vi "IFC.vi"(0 "System no.":i32=1 min=1 step=1, 2 "Interface parameter":string[](array[string]), 3 "Parameter value":string[](array[string]), 5 "error in":errorcluster) -> (19 "error out":errorcluster)   [LabVIEW 2026]
doc: "Changes the current interface configuration. After IFC is sent, the new interface configuration of the controller becomes active and the host must change the interface configuration too. Settings made with IFC are valid until the controller is powered down. \nTo save them to EPROM and make them the default use IFS instead.\n\nC-884: MACADR cannot be changed with IFC. To change IPADR the use of IFS is recommended instead. \n\nC-885: MACADR cannot be changed with IFC. To change IPADR the use of IFS is recommended instead.\n\nE-517: The current active RS-232 baud rate and GPIB (IEEE 488) address can also be set on the E-517 front panel in the COMMUNICATION display screen. This screen can be accessed by the trackball. The front panel settings interdepend with the interface parameter settings set with IFC. See E-517 user manual for details.\n\nE-709: Use IFC to change baud rate settings only.\n\nE-712, E-725, E-727, E-753, E-754, E-871, E-872, E-873, E-874: Use IFC to change baud rate settings only, for all other settings use IFS instead."
panel:
  # "Changes the current InterFace Configuration. After IFC is sent, the new interface\nconfiguration of the controller becomes active and the host must change the interface\nconfiguration too. Settings made with IFC are valid until the controller is powered down. \nTo save them to EPROM and make them the default use IFS instead."
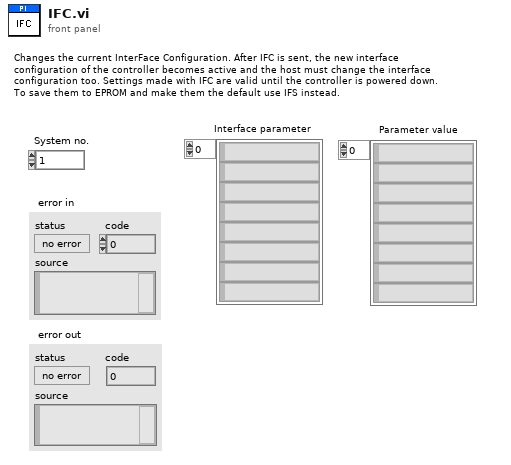
[diagram p1: front panel]
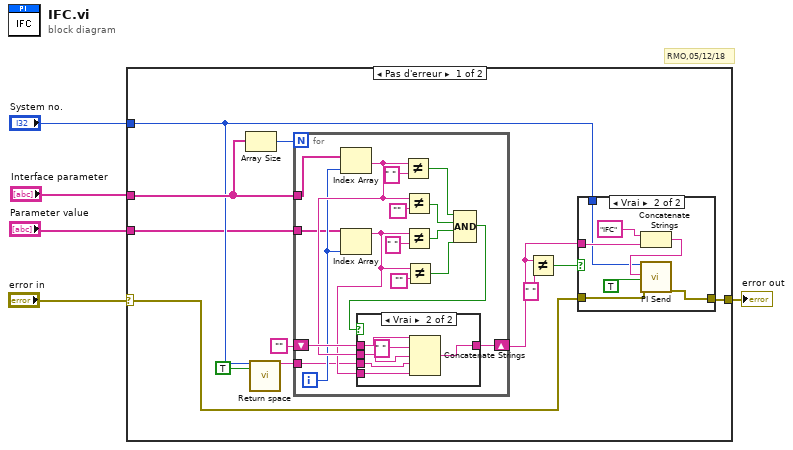
[diagram p0: block diagram]
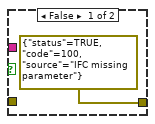
[diagram p2: hidden frame]
diagram:
  # "RMO,05/12/18"
  n1 = case shown="Pas d'erreur" "error in" {
    selector: "error in" -> [w6 w50]
    tunnel: "Interface parameter" -> [w17 _]
    tunnel: [w8 w50] -> w4
    tunnel: "Parameter value" -> [w15 _]
    tunnel: "System no." -> [w16 _]
    frame No Error {
      n2 = Array Size(array=w17) -> (size(s)=w10:i32)
      n3 = call "Return space.vi"("System no."=w16, "With space?"=TRUE) -> ("String out"=w9:string)  [unwired: 17 out]
      n4 = for {
        N: w10 -> [_]
        tunnel: w17 -> [w31]
        shift-right: [w40] -> w12
        shift-left: "" -> [w41]
        tunnel: w15 -> [w29]
        tunnel: w9 -> [w26]
        i -> [w30]
        n5 = Index Array(array=w31, index=w30) -> (element=w39:string)
        n6 = Index Array(array=w29, index=w30) -> (element=w28:string)
        n7 = Not Equal?(x=w39, y=" ") -> (x != y?=w35:bool)
        n8 = Not Equal?(x=w39, y="") -> (x != y?=w34:bool)
        n9 = Not Equal?(x=w28, y=" ") -> (x != y?=w33:bool)
        n10 = Not Equal?(x=w28, y="") -> (x != y?=w32:bool)
        n11 = Compound Arithmetic op=AND(w35, w34, w33, w32) -> (w27:bool)
        n12 = case shown="Vrai" w27 {
          tunnel: w41 -> [w43 w49]
          tunnel: w39 -> [_ w46]
          tunnel: [w43 w48] -> w40
          tunnel: w28 -> [_ w45]
          tunnel: w26 -> [_ w44]
          frame False {
          }
          frame True {
            n13 = Concatenate Strings(w49, " ", w46, w44, w45) -> (w48:string)
          }
        }
      }
      n14 = Not Equal?(x=w12, y=" ") -> (x != y?=w11:bool)
      n15 = case shown="Vrai" w11 {
        tunnel: w12 -> [_ w23]
        tunnel: w6 -> [_ w21]
        tunnel: w16 -> [_ w20]
        tunnel: [errorcluster {"status"=TRUE, "code"=100, "source"="IFC missing parameter"} ("error out") w19] -> w8
        frame False {
        }
        frame True {
          n16 = Concatenate Strings("IFC", w23) -> (w22:string)
          n17 = call "PI Send.vi"("System no."=w20, "String to send"=w22, "Attach termination char.?"=TRUE ("Attach Linefeed?"), "error in"=w21) -> ("error out"=w19:errorcluster)  [unwired: 2 in, 13 out]
        }
      }
    }
    frame Error {
    }
  }
  "error out" <- w4
